vi "VideoWriter Open.vi"   [LabVIEW 2020, in "OpenLvVision_OpenCv.lvlib" / "VideoWriter.lvclass"]
doc: "Initializes or reinitializes video writer."
uses:
  VideoWriter.lvclass
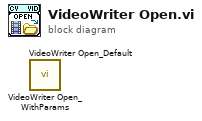
[diagram p0: block diagram]
diagram:
  n1 = call "VideoWriter Open_WithParams.vi"() -> ()  [unwired: 9 in, 3 out]
  n2 = call "VideoWriter Open_Default.vi"() -> ()  [unwired: 9 in, 3 out]
